vi "UI Panel Bounds.vi"(8 "error in (no error)":errorcluster, 10 "Front Panel Window:Panel Bounds":T1, 11 "MainUI in":refnum<class "UI_Top_Customer.lvclass">) -> (0 "error out":errorcluster, 3 "MainUI out":refnum<class "UI_Top_Customer.lvclass">)   [LabVIEW 2021, in "UI_Top_Customer.lvclass"]
uses:
  UI_Top_Customer.lvclass
  UI_Top_Customer.lvclass/UI_Top_Customer.ctl
  <vilib>/Utility/miscctls.llb/LVRectTypeDef.ctl
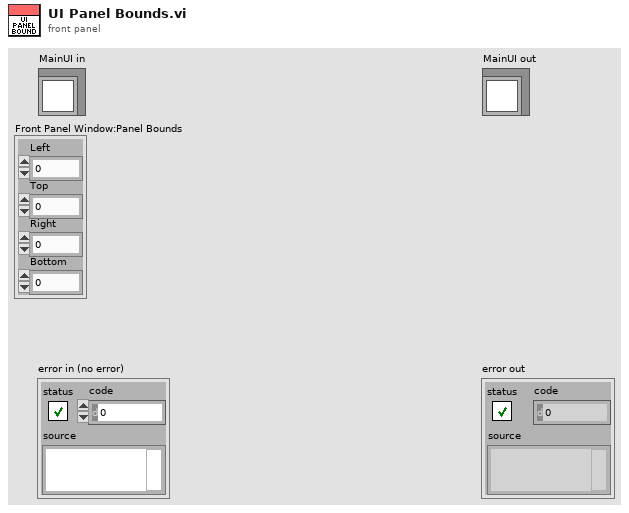
[diagram p1: front panel]
types:
  T1 = typedef "LVRectTypeDef.ctl" = cluster{"Left":i16, "Top":i16, "Right":i16, "Bottom":i16}
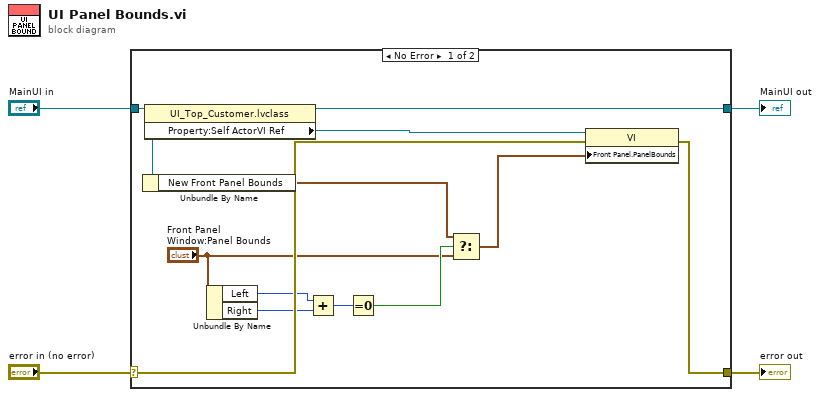
[diagram p0: block diagram]
diagram:
  n1 = case shown="No Error" "error in (no error)" {
    selector: "error in (no error)" -> [w14 w18]
    tunnel: [w13 w18] -> w3
    tunnel: [w15 w17] -> w1
    tunnel: "MainUI in" -> [w9 w17]
    frame No Error {
      n2 = Unbundle By Name(w9) -> ("New Front Panel Bounds"=w7:T1)
      n3 = property class="UI_Top_Customer.lvclass"(reference=w9) -> (reference out=w15:refnum<class "UI_Top_Customer.lvclass">, "Property:Self ActorVI Ref"=w16:refnum<vi>)  [unwired: 1 in, 1 out]
      n4 = Unbundle By Name("Front Panel Window:Panel Bounds") -> ("Left"=w12:i16, "Right"=w11:i16)
      n5 = Add(x=w12, y=w11) -> (x+y=w10:i16)
      n6 = Equal To 0?(x=w10) -> (x = 0?=w8:bool)
      n7 = Select(t=w7, s=w8, f="Front Panel Window:Panel Bounds") -> (s? t:f=w5:T1)
      n8 = property class="VI"(reference=w16, error in=w14, "Front Panel.PanelBounds"=w5) -> (error out=w13:errorcluster)  [unwired: 1 out]
    }
    frame Error {
    }
  }
  "error out" <- w3
  "MainUI out" <- w1
